vi "Komponenten setzen mit Konzentration.vi"(8 "error in (no error)":errorcluster caption="Fehler (Eingang, kein Fehler)", 10 "Komponenten":T1[](array[typedef]) {"Konzentration IST" format="%#.4f"; "Genauigkeit" format="%#.1f"}) -> (0 "error out":errorcluster caption="Fehler (Ausgang)", 1 "Konzentrationen":dbl[](array[numeric]), 2 "Index":i32[](array[numeric]), 3 "found":bool[](array[boolean]), 5 "Indizes":i32[](array[numeric]))   [LabVIEW 2020, in "System Einstellungen V2.lvlib"]
uses:
  System Einstellungen V2.lvlib
  Gasflaschenkomponente.ctl
  FT-IR/FGV FT-IR Gasliste Aktionen.ctl
  FT-IR/FT-IR.lvlib
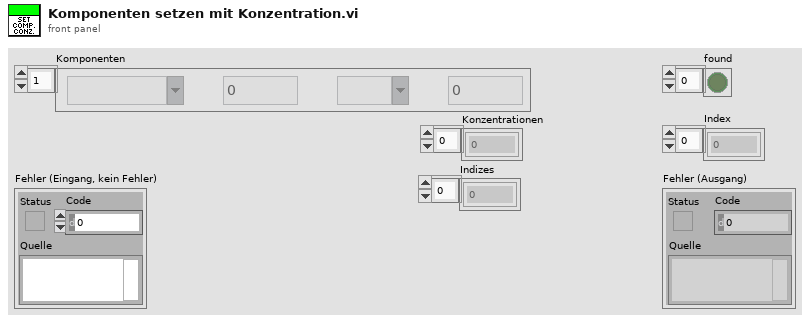
[diagram p1: front panel]
types:
  T1 = typedef "System Einstellungen V2.lvlib/Gasflaschenkomponente.ctl" = cluster{"Gasauswahl":string, "Konzentration IST":dbl, "Einheit":string, "Genauigkeit":dbl}
  T2 = typedef "FT-IR.lvlib/FGV FT-IR Gasliste Aktionen.ctl" = enum16{"lesen", "Gasliste FT-IR", "Gasliste ausgelesen", "laden", "speichern", "löschen"}
  T3 = typedef "String - Ausgabefeld.ctl" = string
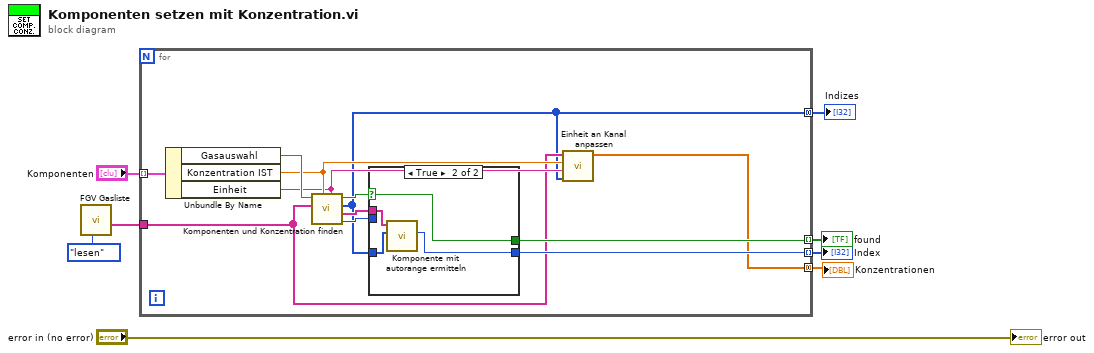
[diagram p0: block diagram]
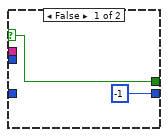
[diagram p2: hidden frame]
diagram:
  n1 = call "FGV Gasliste.vi"("Aktionen"=FGV_FT-IR_Gasliste_Aktionen."lesen") -> ("Aktuelle Gasliste gesamt"=w5:T3[])  [unwired: 8 in, 2 out]
  n2 = for {
    tunnel: w5 -> [w11]
    tunnel: "Komponenten" -> [w20] mode=indexing
    tunnel: [w19] -> w4 mode=indexing
    tunnel: [w13] -> w3 mode=indexing
    tunnel: [w9] -> w2 mode=concatenating
    tunnel: [w10] -> w1 mode=concatenating
    n3 = Unbundle By Name(w20) -> ("Gasauswahl"=w17:string, "Konzentration IST"=w14:dbl, "Einheit"=w12:string)
    n4 = call "Komponenten und Konzentration finden.vi"("Einheit"=w12, "Konzentration"=w14, "Aktuelle Gasliste gesamt"=w11, "String"=w17) -> ("biggest Channel"=w15:i32, "Gasliste"=w16:string[], "Indizes"=w10:i32[], "Channel found"=w18:bool)  [unwired: 3 in, 1 out]
    n5 = case shown="True" w18 {
      selector: w18 -> [w22 w26]
      tunnel: w10 -> [_ w25]
      tunnel: [w22 w26] -> w19
      tunnel: [-1 ("Index") w23] -> w13
      tunnel: w16 -> [_ w24]
      tunnel: w15 -> [_ _]
      frame False {
      }
      frame True {
        n6 = call "Komponente mit autorange ermitteln.vi"("Indizes"=w25, "Gasliste"=w24) -> ("Index"=w23:i32)  [unwired: 8 in, 1 out]
      }
    }
    n7 = call "Einheit an Kanal anpassen.vi"("Indizes"=w10, "Einheit"=w12, "Konzentration IST"=w14, "Aktuelle Gasliste gesamt"=w11) -> ("Konzentrationen"=w9:dbl[])  [unwired: 7 in]
  }
  "found" <- w4
  "Index" <- w3
  "Konzentrationen" <- w2
  "Indizes" <- w1
  "error out" <- "error in (no error)"
